vi "PM100D-GetSetRng.vi"(8 "error in (no error)":errorcluster, 10 "Unit":string, 11 "VISA Refnum in":refnum<visa-resource-name>) -> (0 "error out":errorcluster, 2 "Range":dbl, 3 "lblRange":string)   [LabVIEW 2011]
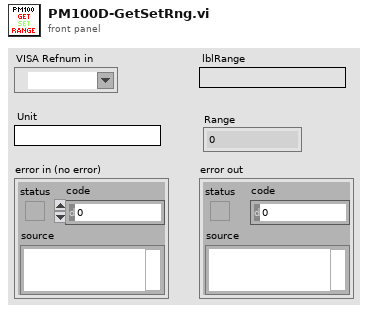
[diagram p1: front panel]
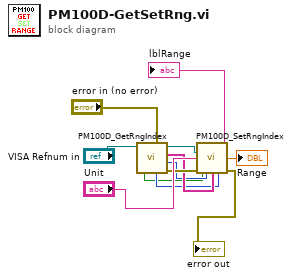
[diagram p0: block diagram]
diagram:
  n1 = call "PM100D_GetRngIndex.vi"("error in (no error)"="error in (no error)", "VISA in"="VISA Refnum in") -> ("error out"=w7:errorcluster, "SensType"=w4:i32, "Rng_Array"=w5:string[], "dup VISA session"=w6:refnum<visa-resource-name>, "IndexOut"=w3:i32, "AutoOut"=w2:bool)  [unwired: 4 in]
  n2 = call "PM100D_SetRngIndex.vi"("VISAin"=w6, "Unit"="Unit", "AUTO"=w2, "error in"=w7, "SensType"=w4, "Rng_Array"=w5, "Index"=w3) -> ("lblRange"=→"lblRange":string, "Numeric 2"=→"Range":dbl, "error out 2"=→"error out":errorcluster)  [unwired: 4 in, 2 out]
